vi "MGI Bezier Scalar.vi"(1 "u":sgl format="%.2f", 2 "k":i32=1, 3 "Bezier Control Points[]":sgl[](array[numeric]) format="%.2f") -> (0 "y":sgl format="%.2f")   [LabVIEW 2020]
doc: "Compute a Bezier point given an array of control points, the index of the start of the block of 4 points to be used, and the desired 0-1 value.\n\nAuthored by David A. Moore\nsupport@mooregoodideas.com\nwww.mooregoodideas.com\n\nCopyright (c) 2010, Moore Good Ideas, Inc.\n\nAll rights reserved.\n\nRedistribution and use in source and binary forms, with or without modification, are permitted provided that the following conditions are met:\n\n * Redistributions of source code must retain the above copyright notice, this list of conditions and the following disclaimer.\n * Redistributions in binary form must reproduce the above copyright notice, this list of conditions and the following disclaimer in the documentation and/or other materials provided with the distribution.\n * Neither the name of Moore Good Ideas, Inc. nor the names of its contributors may be used to endorse or promote products derived from this software without specific prior written permission.\n\nTHIS SOFTWARE IS PROVIDED BY THE COPYRIGHT HOLDERS AND CONTRIBUTORS \"AS IS\" AND ANY EXPRESS OR IMPLIED WARRANTIES, INCLUDING, BUT NOT LIMITED TO, THE IMPLIED WARRANTIES OF MERCHANTABILITY AND FITNESS FOR A PARTICULAR PURPOSE ARE DISCLAIMED. IN NO EVENT SHALL THE COPYRIGHT OWNER OR CONTRIBUTORS BE LIABLE FOR ANY DIRECT, INDIRECT, INCIDENTAL, SPECIAL, EXEMPLARY, OR CONSEQUENTIAL DAMAGES (INCLUDING, BUT NOT LIMITED TO, PROCUREMENT OF SUBSTITUTE GOODS OR SERVICES; LOSS OF USE, DATA, OR PROFITS; OR BUSINESS INTERRUPTION) HOWEVER CAUSED AND ON ANY THEORY OF LIABILITY, WHETHER IN CONTRACT, STRICT LIABILITY, OR TORT (INCLUDING NEGLIGENCE OR OTHERWISE) ARISING IN ANY WAY OUT OF THE USE OF THIS SOFTWARE, EVEN IF ADVISED OF THE POSSIBILITY OF SUCH DAMAGE."
uses:
  <userlib>/_MGI/Bezier/MGI Bezier Weights/MGI Bezier Weights (SGL).vi
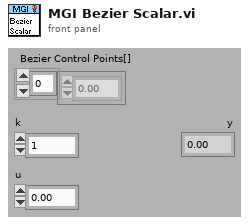
[diagram p1: front panel]
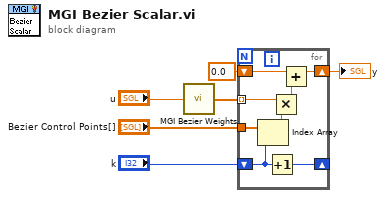
[diagram p0: block diagram]
diagram:
  n1 = call-poly <userlib>:"MGI Bezier Weights.vi"("u"="u") -> ("Bezier Weights"=w5:sgl[])
  n2 = for {
    tunnel: w5 -> [w10] mode=indexing
    tunnel: "Bezier Control Points[]" -> [w14]
    shift-right: [w12] -> _
    shift-left: "k" -> [w13]
    shift-right: [w8] -> w1
    shift-left: sgl 0.0 -> [w7]
    n3 = Index Array(array=w14, index=w13) -> (element=w11:sgl)
    n4 = Increment(x=w13) -> (x+1=w12:i32)
    n5 = Multiply(x=w10, y=w11) -> (x*y=w9:sgl)
    n6 = Add(x=w7, y=w9) -> (x+y=w8:sgl)
  }
  "y" <- w1
